vi "Display.vi"(8 "Error In":errorcluster, 11 "reference in":refnum<class "RealImage.lvclass">) -> (0 "Error Out":errorcluster, 3 "reference out":refnum<class "RealImage.lvclass">)   [LabVIEW 2020, in "RealImage.lvclass"]
uses:
  RealImage.lvclass
  Console_class/Console.lvclass
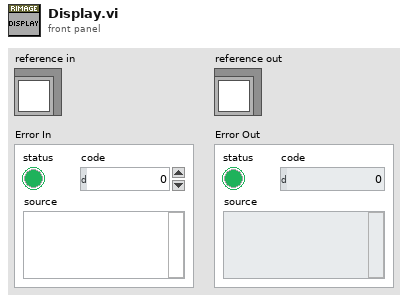
[diagram p1: front panel]
types:
  T1 = typedef "RealImage.lvclass/ObjectAttributes.ctl" = cluster{"_fileName":string}
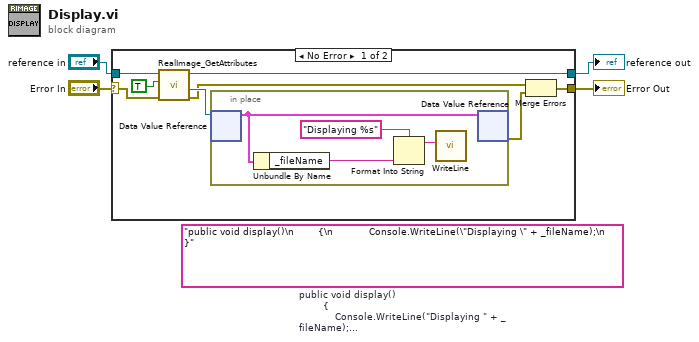
[diagram p0: block diagram]
diagram:
  (unwired) "public void display()\n        {\n            Console.WriteLine(\"Displaying \" + _fileName);\n        }"  # public void display()         {             Console.WriteLine("Displaying " + _fileName);         }
  n1 = case shown="No Error" "Error In" {
    selector: "Error In" -> [w11 w18]
    tunnel: [w8 w18] -> w3
    tunnel: [w9 w17] -> w1
    tunnel: "reference in" -> [w12 w17]
    frame No Error {
      n2 = call "RealImage_GetAttributes.vi"("error in (no error)"=w11, "OnlyGetDvrReference(False)"=TRUE, "reference in"=w12) -> ("error out"=w6:errorcluster, "DataRef"=w7:refnum<data-value>, "reference out"=w9:refnum<class "RealImage.lvclass">)  [unwired: 5 in, 1 out]
      n3 = in-place {
        n4 = in-place-dvr #1(w7) -> (w16:T1)  [unwired: 1 out]
        n5 = Unbundle By Name(w16) -> ("_fileName"=w14:string)
        n6 = Format Into String(format string="Displaying %s", w14) -> (resulting string=w13:string)  [unwired: 2 in, 1 out]
        n7 = call "WriteLine.vi"("ConsoleText"=w13) -> ()  [unwired: 10 in, 1 out]
        n8 = in-place-dvr #1(w16) -> (w10:errorcluster)  [unwired: 1 out]
      }
      n9 = Merge Errors(w6, w10) -> (w8:errorcluster)
    }
    frame Error {
    }
  }
  "Error Out" <- w3
  "reference out" <- w1
